vi "XY Graph Plot Interpolation.vi"(8 "error in (no error)":errorcluster, 10 "Active Plot":u32, 11 "XYGraph in":T1) -> (0 "error out":errorcluster, 2 "Bin Location":T2, 3 "Plot Interpolation":u8)   [LabVIEW 2019]
uses:
  Histograms/Histogram Bin Position.ctl
  XY Graph Refnum.ctl
  XY Graph Add-Ons.lvlib
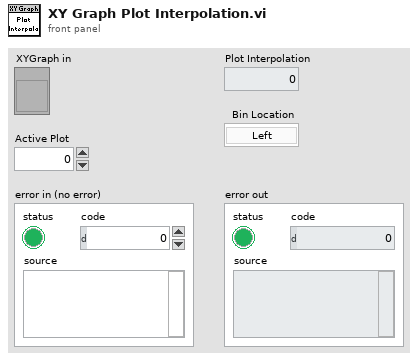
[diagram p1: front panel]
types:
  T1 = typedef "XY Graph Add-Ons.lvlib/XY Graph Refnum.ctl" = refnum<vi>
  T2 = typedef "Histogram Bin Position.ctl" = enum16{"Left", "Center", "Right"}
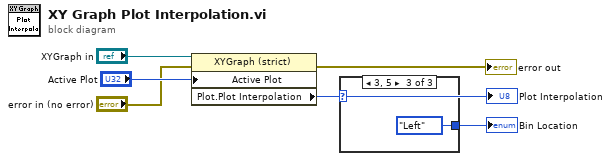
[diagram p0: block diagram]
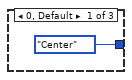
[diagram p2: hidden frame]
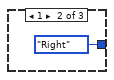
[diagram p3: hidden frame]
diagram:
  n1 = property class="XYGraph (strict)"(reference="XYGraph in", error in="error in (no error)", "Active Plot"="Active Plot") -> (error out=→"error out":errorcluster, "Plot.Plot Interpolation"=w5:u8)  [unwired: 1 out]
  "Plot Interpolation" <- w5
  n2 = case shown="3, 5" w5 {
    tunnel: [Histogram_Bin_Position."Center" ("Bin Location") Histogram_Bin_Position."Right" ("Bin Location") Histogram_Bin_Position."Left" ("Bin Location")] -> w6
    frame 0, Default {
    }
    frame 1 {
    }
    frame 3, 5 {
    }
  }
  "Bin Location" <- w6
